vi "Create User Event.vi"(8 "error in (no error)":errorcluster caption="에러 입력(에러 없음)") -> (0 "error out":errorcluster caption="에러 출력", 3 "User Event":refnum<user-event>)   [LabVIEW 2018, in "User Event.lvlib"]
doc: "메시지 핸들링 루프에서 이벤트 루프를 정지하는데 사용되는 불리언 사용자 이벤트를 생성합니다."
uses:
  User Event.lvlib
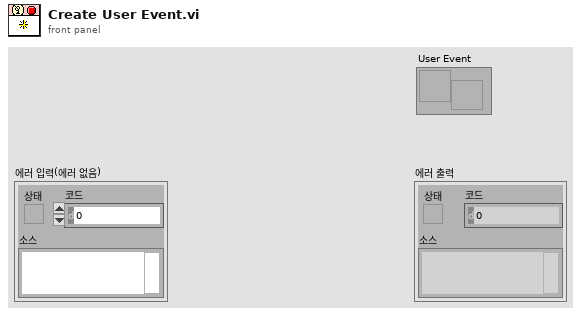
[diagram p1: front panel]
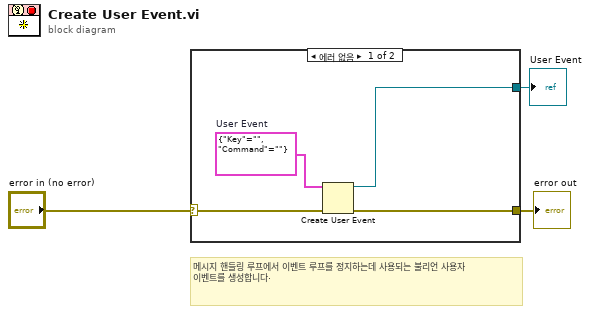
[diagram p0: block diagram]
diagram:
  # "메시지 핸들링 루프에서 이벤트 루프를 정지하는데 사용되는 불리언 사용자 이벤트를 생성합니다."
  n1 = case shown="에러 없음" "error in (no error)" {
    selector: "error in (no error)" -> [w7 w8]
    tunnel: [w5 _] -> w1
    tunnel: [w6 w8] -> w3
    frame No Error {
      w4 = cluster{"Key":string, "Command":string} {"Key"="", "Command"=""}  # User Event
      n2 = Create User Event(user event datatype=w4, error in=w7) -> (user event=w5:refnum<user-event>, error out=w6:errorcluster)
    }
    frame Error {
    }
  }
  "error out" <- w3
  "User Event" <- w1
